vi "ChannelsToLog.vi"(11 "Sensor Info":string[][](array[string])) -> (2 "ReportHeader":string[](array[string]), 3 "ChannelTag":string[](array[string]))   [LabVIEW 2018, in "File IO.lvlib"]
uses:
  File IO.lvlib
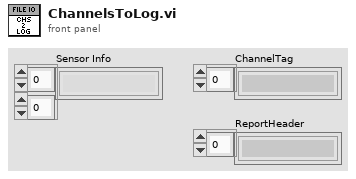
[diagram p1: front panel]
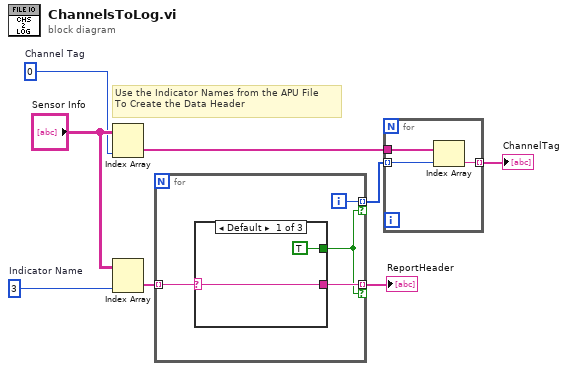
[diagram p0: block diagram]
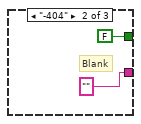
[diagram p2: hidden frame]
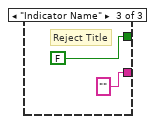
[diagram p3: hidden frame]
diagram:
  w4 = 0  # Channel Tag
  w1 = 3  # Indicator Name
  # "Use the Indicator Names from the APU File\nTo Create the Data Header"
  n1 = Index Array(array="Sensor Info", index (col)=w4) -> (element=w5:string[])  [unwired: 1 in]
  n2 = Index Array(array="Sensor Info", index (col)=w1) -> (element=w2:string[])  [unwired: 1 in]
  n3 = for {
    tunnel: w2 -> [w12] mode=indexing
    tunnel: [w11] -> w3 mode=indexing if=w9
    tunnel: [w10] -> w7 mode=indexing if=w9
    i -> [w10]
    n4 = case shown="Default" w12 {
      selector: w12 -> [w14 _ _]
      tunnel: [w14 "" ""] -> w11
      tunnel: [TRUE FALSE FALSE] -> w9
      frame Default {
      }
      frame "-404" {
        # "Blank"
      }
      frame "Indicator Name" {
        # "Reject Title"
      }
    }
  }
  "ReportHeader" <- w3
  n5 = for {
    tunnel: w5 -> [w21]
    tunnel: [w20] -> w8 mode=indexing
    tunnel: w7 -> [w19] mode=indexing
    n6 = Index Array(array=w21, index=w19) -> (element=w20:string)
  }
  "ChannelTag" <- w8
